vi "BRig_dataExp_SolenoidProb_L.vi"() -> (2 "output_SolenoidProbability_L":i32)   [LabVIEW 2014]
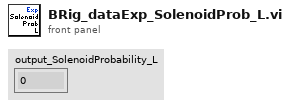
[diagram p1: front panel]
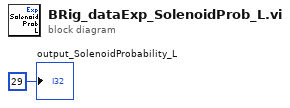
[diagram p0: block diagram]
diagram:
  "output_SolenoidProbability_L" <- 29 ("output_iBlock")
